vi "curv calibrarrion.vi"(0 "sensor1 array":dbl[](array[numeric]), 1 "sensor2 array":dbl[](array[numeric]), 2 "sensor2 array":dbl[](array[numeric]), 3 "sensor data array":dbl[](array[numeric])) -> (14 "sensor1 array out":dbl[](array[numeric]), 15 "sensor2 array out":dbl[](array[numeric]), 16 "sensor3 array out":dbl[](array[numeric]), 17 "This VI":refnum<vi>)   [LabVIEW 2019]
panel:
  out "curv":dbl
  out "sensor1 dis 3":dbl
  out "sensor1 dis 2":dbl
  out "sensor1 dis":dbl
  in  "curv calculate":bool
  in  "get distance":bool
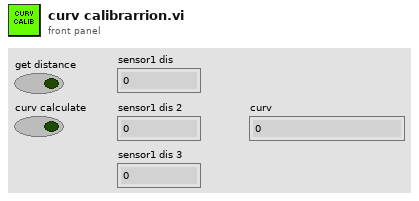
[diagram p1: front panel]
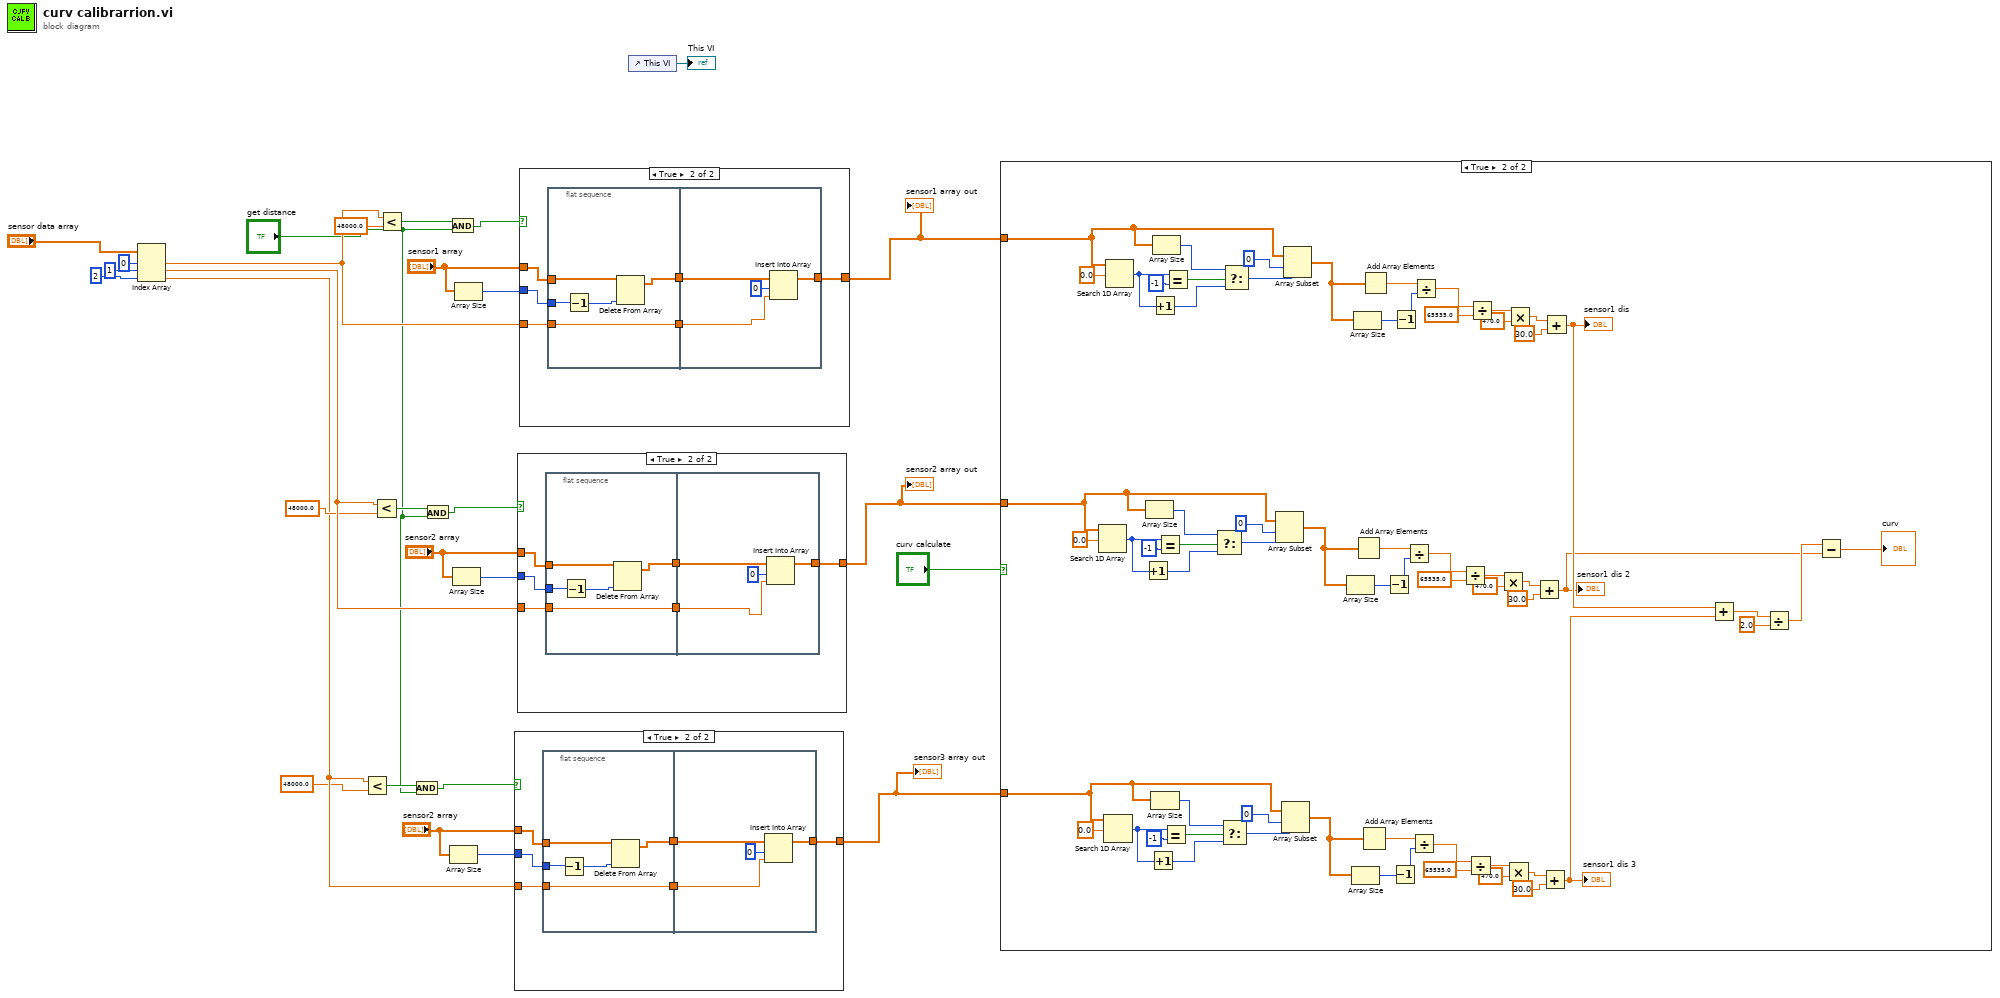
[diagram p0: block diagram]
diagram:
  n1 = Index Array(array="sensor data array", index #1=0 ("index"), index #2=1 ("index"), index #3=2 ("index")) -> (element #1=w21:dbl, element #2=w19:dbl, element #3=w17:dbl)
  n2 = Less?(x=w17, y=48000.0) -> (x < y?=w11:bool)
  n3 = Less?(x=w19, y=48000.0) -> (x < y?=w12:bool)
  n4 = Less?(x=w21, y=48000.0) -> (x < y?=w15:bool)
  n5 = And(x=w11, y="get distance") -> (x .and. y?=w9:bool)
  n6 = And(x=w12, y="get distance") -> (x .and. y?=w13:bool)
  n7 = And(x=w15, y="get distance") -> (x .and. y?=w14:bool)
  n8 = Array Size(array="sensor2 array") -> (size(s)=w26:i32)
  n9 = Array Size(array="sensor2 array") -> (size(s)=w27:i32)
  n10 = Array Size(array="sensor1 array") -> (size(s)=w28:i32)
  n11 = case shown="True" w9 {
    tunnel: "sensor2 array" -> [w29 w35]
    tunnel: w26 -> [_ w34]
    tunnel: [w29 w32] -> w5
    tunnel: w17 -> [_ w31]
    frame False {
    }
    frame True {
      n12 = flat-sequence {
        tunnel: w35 -> [w40]
        tunnel: w34 -> [w39]
        tunnel: [w37] -> w33
        tunnel: w31 -> [w36]
        tunnel: [w36] -> w30
        tunnel: [w44] -> w32
        tunnel: w33 -> [w43]
        tunnel: w30 -> [w41]
        frame #0 {
          n13 = Decrement(x=w39) -> (x-1=w38:i32)
          n14 = Delete From Array(array=w40, index=w38) -> (array with subset deleted=w37:dbl[])  [unwired: 1 in, 1 out]
        }
        frame #1 {
          n15 = Insert Into Array(array=w43, index=0, new element=w41) -> (w44:dbl[])
        }
      }
    }
  }
  "sensor3 array out" <- w5
  n16 = case shown="True" w13 {
    tunnel: "sensor2 array" -> [w45 w51]
    tunnel: w27 -> [_ w50]
    tunnel: [w45 w48] -> w6
    tunnel: w19 -> [_ w46]
    frame False {
    }
    frame True {
      n17 = flat-sequence {
        tunnel: w51 -> [w56]
        tunnel: w50 -> [w55]
        tunnel: [w53] -> w49
        tunnel: [w52] -> w47
        tunnel: w46 -> [w52]
        tunnel: [w60] -> w48
        tunnel: w49 -> [w59]
        tunnel: w47 -> [w57]
        frame #0 {
          n18 = Decrement(x=w55) -> (x-1=w54:i32)
          n19 = Delete From Array(array=w56, index=w54) -> (array with subset deleted=w53:dbl[])  [unwired: 1 in, 1 out]
        }
        frame #1 {
          n20 = Insert Into Array(array=w59, index=0, new element=w57) -> (w60:dbl[])
        }
      }
    }
  }
  "sensor2 array out" <- w6
  n21 = case shown="True" w14 {
    tunnel: "sensor1 array" -> [w61 w67]
    tunnel: w28 -> [_ w66]
    tunnel: [w61 w64] -> w7
    tunnel: w21 -> [_ w62]
    frame False {
    }
    frame True {
      n22 = flat-sequence {
        tunnel: w67 -> [w72]
        tunnel: w66 -> [w71]
        tunnel: [w69] -> w65
        tunnel: [w68] -> w63
        tunnel: w62 -> [w68]
        tunnel: [w76] -> w64
        tunnel: w65 -> [w75]
        tunnel: w63 -> [w73]
        frame #0 {
          n23 = Decrement(x=w71) -> (x-1=w70:i32)
          n24 = Delete From Array(array=w72, index=w70) -> (array with subset deleted=w69:dbl[])  [unwired: 1 in, 1 out]
        }
        frame #1 {
          n25 = Insert Into Array(array=w75, index=0, new element=w73) -> (w76:dbl[])
        }
      }
    }
  }
  "sensor1 array out" <- w7
  n26 = control-ref of="This VI"() -> (→"This VI":refnum<vi>)
  n27 = case shown="True" "curv calculate" {
    tunnel: w7 -> [_ w139]
    tunnel: w6 -> [_ w137]
    tunnel: w5 -> [_ w135]
    frame False {
    }
    frame True {
      n28 = Search 1D Array(1D array=w137, element=0.0) -> (index of element=w104:i32)  [unwired: 1 in]
      n29 = Search 1D Array(1D array=w135, element=0.0) -> (index of element=w87:i32)  [unwired: 1 in]
      n30 = Search 1D Array(1D array=w139, element=0.0) -> (index of element=w121:i32)  [unwired: 1 in]
      n31 = Increment(x=w104) -> (x+1=w103:i32)
      n32 = Array Size(array=w137) -> (size(s)=w138:i32)
      n33 = Increment(x=w87) -> (x+1=w86:i32)
      n34 = Increment(x=w121) -> (x+1=w120:i32)
      n35 = Array Size(array=w135) -> (size(s)=w136:i32)
      n36 = Array Size(array=w139) -> (size(s)=w140:i32)
      n37 = Equal?(x=w104, y=-1) -> (x = y?=w105:bool)
      n38 = Equal?(x=w87, y=-1) -> (x = y?=w88:bool)
      n39 = Equal?(x=w121, y=-1) -> (x = y?=w122:bool)
      n40 = Select(t=w138, s=w105, f=w103) -> (s? t:f=w102:i32)
      n41 = Select(t=w136, s=w88, f=w86) -> (s? t:f=w85:i32)
      n42 = Select(t=w140, s=w122, f=w120) -> (s? t:f=w119:i32)
      n43 = Array Subset(array=w137, index=0, length=w102) -> (w101:dbl[])
      n44 = Array Subset(array=w135, index=0, length=w85) -> (w84:dbl[])
      n45 = Array Subset(array=w139, index=0, length=w119) -> (w118:dbl[])
      n46 = Array Size(array=w101) -> (size(s)=w113:i32)
      n47 = Array Size(array=w84) -> (size(s)=w96:i32)
      n48 = Array Size(array=w118) -> (size(s)=w130:i32)
      n49 = Add Array Elements(numeric array=w101) -> (sum=w112:dbl)
      n50 = Add Array Elements(numeric array=w84) -> (sum=w95:dbl)
      n51 = Add Array Elements(numeric array=w118) -> (sum=w129:dbl)
      n52 = Decrement(x=w113) -> (x-1=w114:i32)
      n53 = Decrement(x=w96) -> (x-1=w97:i32)
      n54 = Decrement(x=w130) -> (x-1=w131:i32)
      n55 = Divide(x=w112, y=w114) -> (x/y=w115:dbl)
      n56 = Divide(x=w95, y=w97) -> (x/y=w98:dbl)
      n57 = Divide(x=w129, y=w131) -> (x/y=w132:dbl)
      n58 = Divide(x=w115, y=65535.0) -> (x/y=w116:dbl)
      n59 = Divide(x=w98, y=65535.0) -> (x/y=w99:dbl)
      n60 = Divide(x=w132, y=65535.0) -> (x/y=w133:dbl)
      n61 = Multiply(x=w116, y=470.0) -> (x*y=w117:dbl)
      n62 = Multiply(x=w99, y=470.0) -> (x*y=w100:dbl)
      n63 = Multiply(x=w133, y=470.0) -> (x*y=w134:dbl)
      n64 = Add(x=w117, y=30.0) -> (x+y=w77:dbl)
      "sensor1 dis 2" <- w77
      n65 = Add(x=w100, y=30.0) -> (x+y=w83:dbl)
      "sensor1 dis 3" <- w83
      n66 = Add(x=w134, y=30.0) -> (x+y=w82:dbl)
      "sensor1 dis" <- w82
      n67 = Add(x=w82, y=w83) -> (x+y=w80:dbl)
      n68 = Divide(x=w80, y=2.0) -> (x/y=w78:dbl)
      n69 = Subtract(x=w78, y=w77) -> (x-y=→"curv":dbl)
    }
  }
